vi "setgrat.vi"(2 "error in (no error)":errorcluster, 3 "Grating":i32=1 min=1 max=2 step=1) -> (0 "error out":errorcluster)   [LabVIEW 2017]
doc: "Selects the grating for monochromator to use\n\nReturns No Eror in error out for success, See Error Codes"
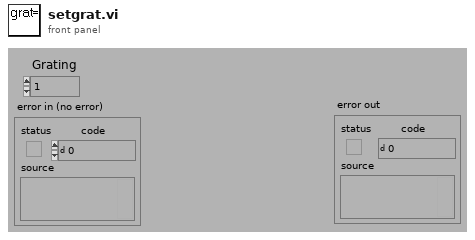
[diagram p1: front panel]
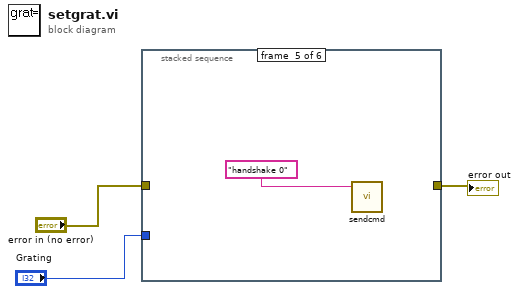
[diagram p0: block diagram]
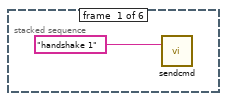
[diagram p2: hidden frame]
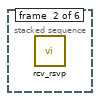
[diagram p3: hidden frame]
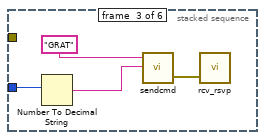
[diagram p4: hidden frame]
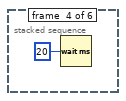
[diagram p5: hidden frame]
diagram:
  n1 = stacked-sequence {
    tunnel: "error in (no error)" -> [_ _ _ _ _ w11]
    tunnel: [_ _ _ _ _ w11] -> w2
    tunnel: "Grating" -> [_ _ w8 _ _ _]
    frame #0 {
      n2 = call "sendcmd.vi"("command in"="handshake 1") -> ()  [unwired: 2 in, 1 out]
    }
    frame #1 {
      n3 = call "rcv_rsvp.vi"() -> ()  [unwired: 2 in, 2 out]
    }
    frame #2 {
      n4 = Number To Decimal String(number=w8) -> (decimal integer string=w6:string)  [unwired: 1 in]
      n5 = call "sendcmd.vi"("parameter"=w6, "command in"="GRAT") -> ("error out"=w5:errorcluster)  [unwired: 1 in]
      n6 = call "rcv_rsvp.vi"("error in (no error)"=w5) -> ()  [unwired: 1 in, 2 out]
    }
    frame #3 {
      n7 = Wait (ms)(milliseconds to wait=u32 20) -> ()  [unwired: 1 out]
    }
    frame #4 {
      n8 = call "sendcmd.vi"("command in"="handshake 0") -> ()  [unwired: 2 in, 1 out]
    }
    frame #5 {
    }
  }
  "error out" <- w2
